vi "Logging Message Loop.vi"(8 "error in (no error)":errorcluster, 9 "Data Notifiers":T1, 10 "Data Queue":refnum<queue>, 11 "Message Queues":T2) -> (0 "error out":errorcluster)   [LabVIEW 2013, in "Logging.lvlib"]
doc: "The message loop subVI to handle messages pertaining to logging data."
uses:
  Logging.lvlib
  support/Message Queue/All Message Queues.ctl
  support/Message Queue/Message Cluster.ctl
  support/Data Notifiers/All Data Notifiers.ctl
  Acquisition/APD Notifier Cluster.ctl
  Piezo/Piezo display.ctl
  XY/XY Display.ctl
  Capacitive/Capacitive Signal Cluster.ctl
  Feedback/Error Signal.ctl
  Logging Configuration.ctl
  Logging State.ctl
  support/Message Queue/Enqueue Message (Single).vi
  <vilib>/Utility/error.llb/Error Cluster From Error Code.vi
  <vilib>/ErrorRing/Error Ring.xnode
  support/Message Queue/Message Queue.lvlib
  Piezo/Piezo.lvlib
  Acquisition/Acquisition.lvlib
  XY/XY.lvlib
  support/Data Notifiers/Data Notifiers.lvlib
  Capacitive/Capacitive.lvlib
  Feedback/Feedback.lvlib
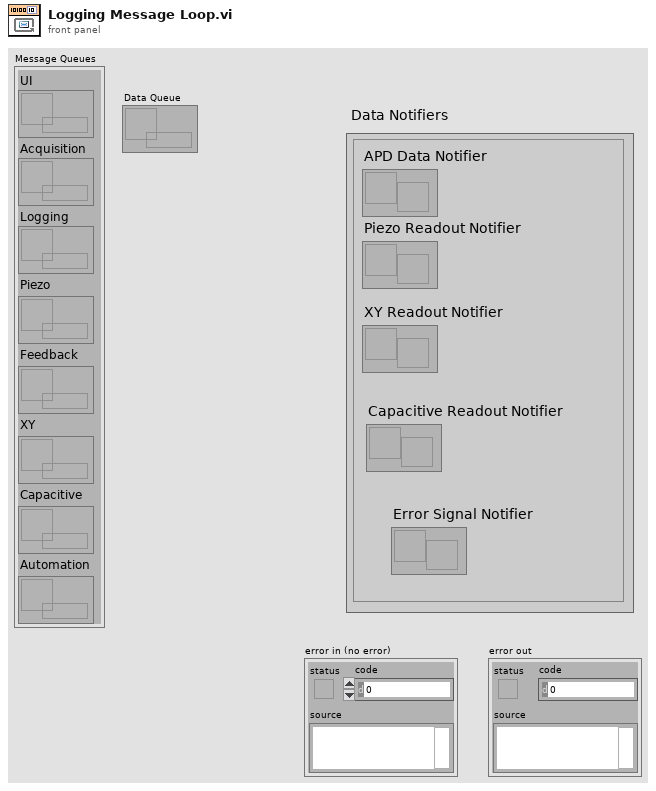
[diagram p1: front panel]
types:
  T1 = typedef "Data Notifiers.lvlib/All Data Notifiers.ctl" = cluster{"APD Data Notifier":refnum<notifier>, "Piezo Readout Notifier":refnum<notifier>, "XY Readout Notifier":refnum<notifier>, "Capacitive Readout Notifier":refnum<notifier>, "Error Signal Notifier":refnum<notifier>}
  T2 = typedef "Message Queue.lvlib/All Message Queues.ctl" = cluster{"UI":refnum<queue>, "Acquisition":refnum<queue>, "Logging":refnum<queue>, "Piezo":refnum<queue>, "Feedback":refnum<queue>, "XY":refnum<queue>, "Capacitive":refnum<queue>, "Automation":refnum<queue>}
  T3 = typedef "Logging.lvlib/Logging State.ctl" = cluster{"State":enum16{"Logging", "Not Logging"}, "Samples to Save":u32, "Start Time":dbl}
  T4 = typedef "Logging.lvlib/Logging Configuration.ctl" = cluster{"Log File Base Path":path, "Max Samples":u32, "File Refnum":refnum<file>, "Log Piezo":bool, "Piezo File Refnum":refnum<file>, "Log Capacitive":bool, "Cap File Refnum":refnum<file>, "Filename":string, "Path where to save":path}
  T5 = cluster{"Value":bool, "Filename":string, "Max. Samp":i32}
  T6 = typedef "Piezo.lvlib/Piezo display.ctl" = cluster{"PiezoPosition":sgl, "Counter Time":i32}
  T7 = typedef "Capacitive.lvlib/Capacitive Signal Cluster.ctl" = cluster{"Readout":sgl, "Time":i32, "Temperature":dbl}
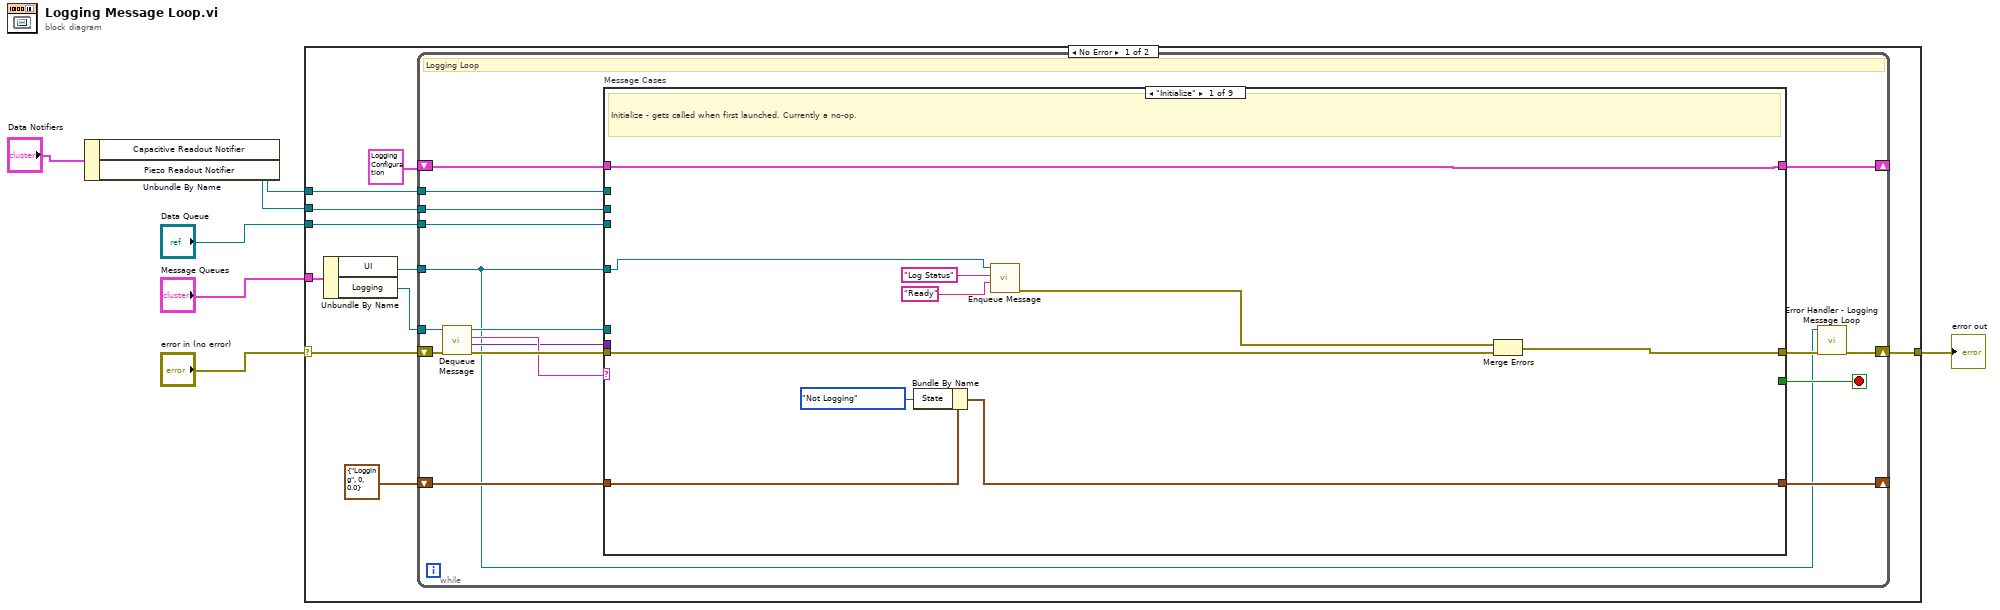
[diagram p0: block diagram]
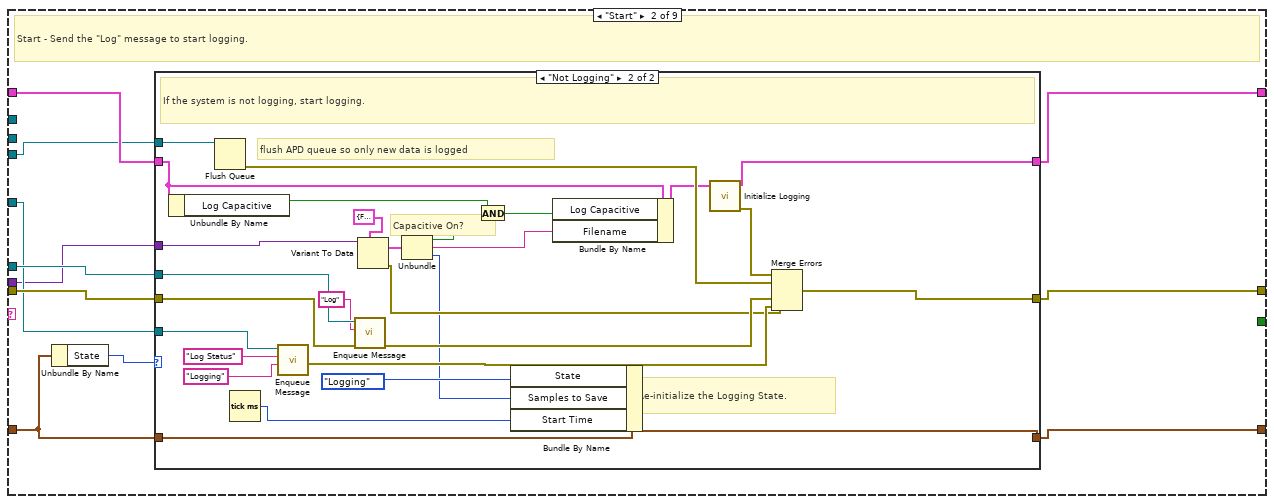
[diagram p2: hidden frame]
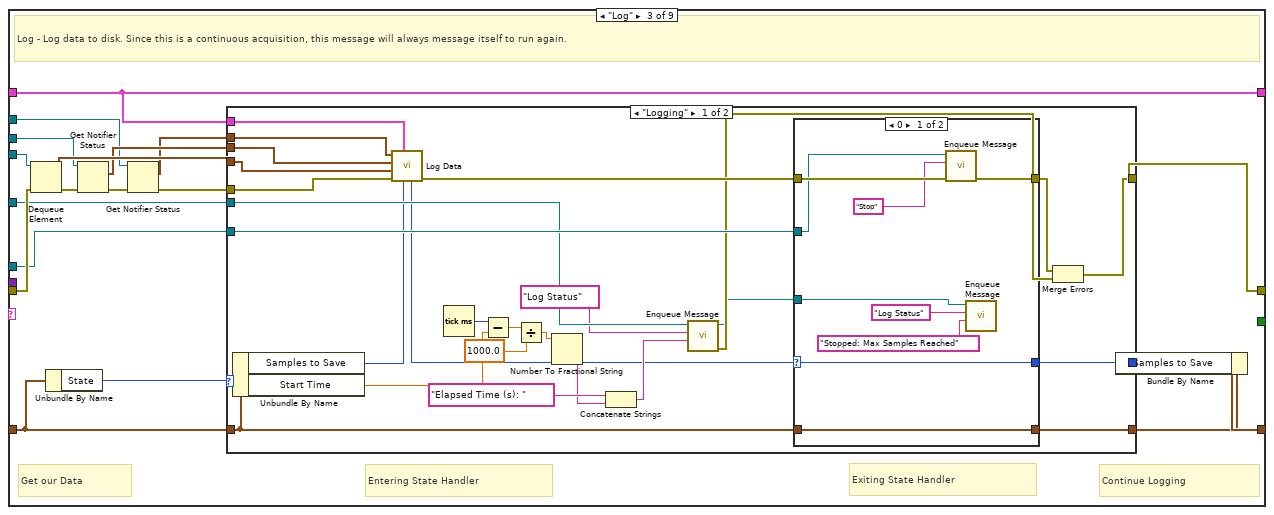
[diagram p4: hidden frame]
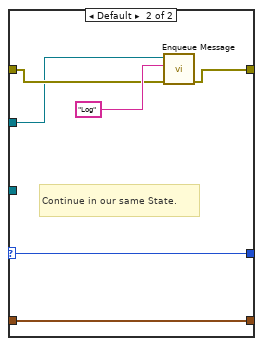
[diagram p5: hidden frame]
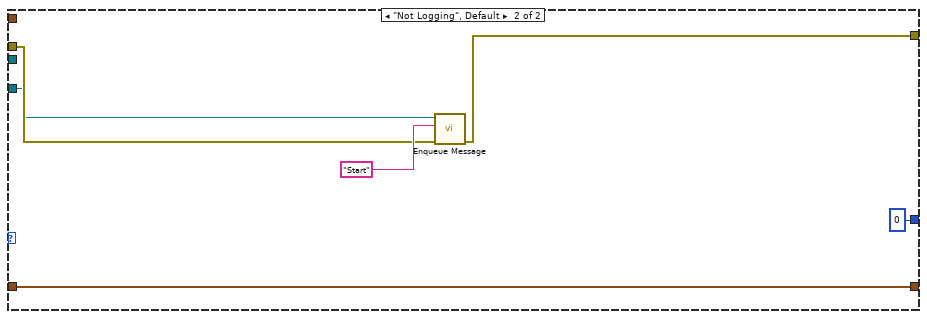
[diagram p6: hidden frame]
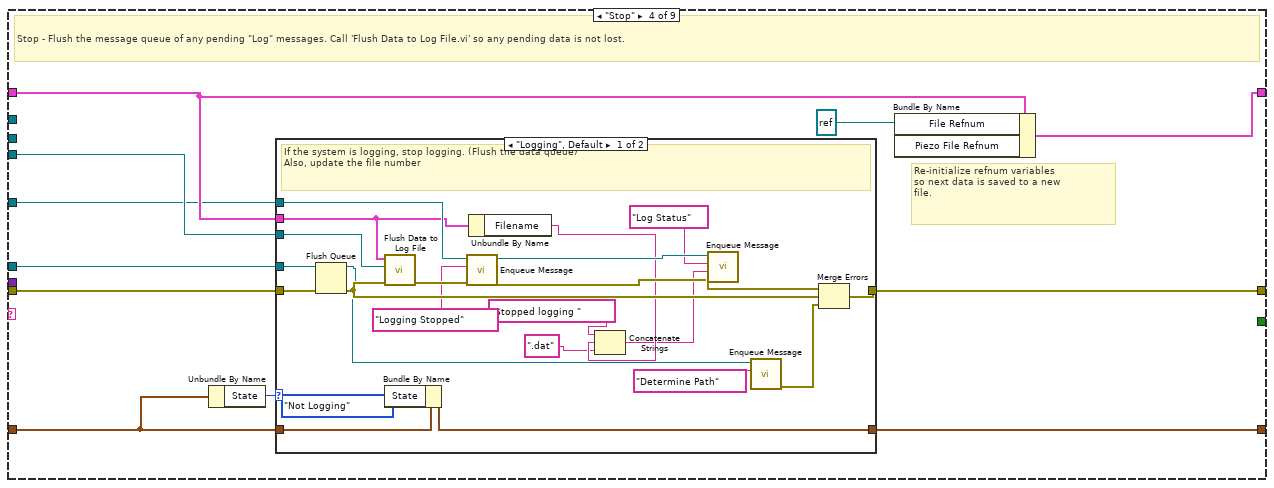
[diagram p7: hidden frame]
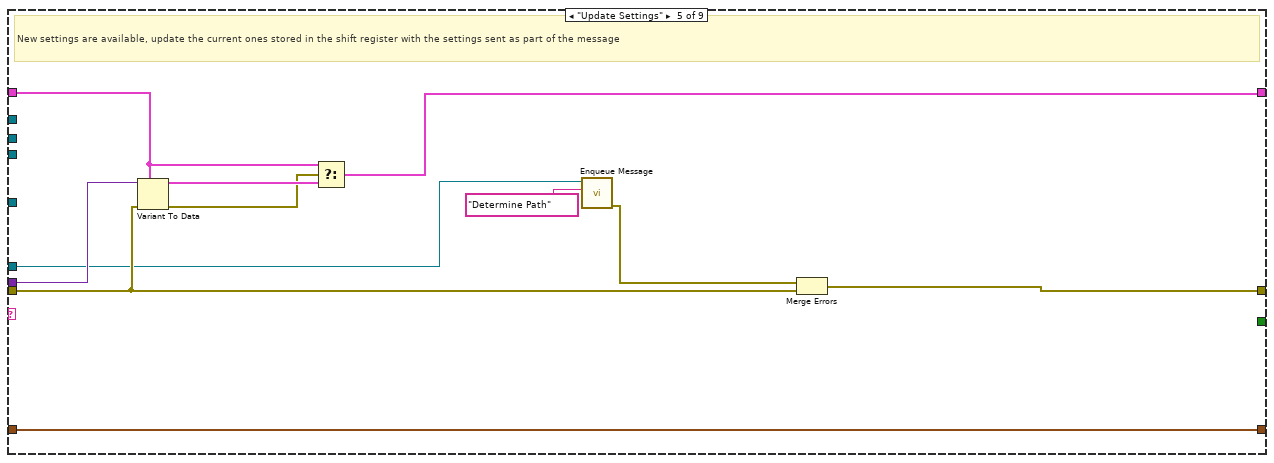
[diagram p9: hidden frame]
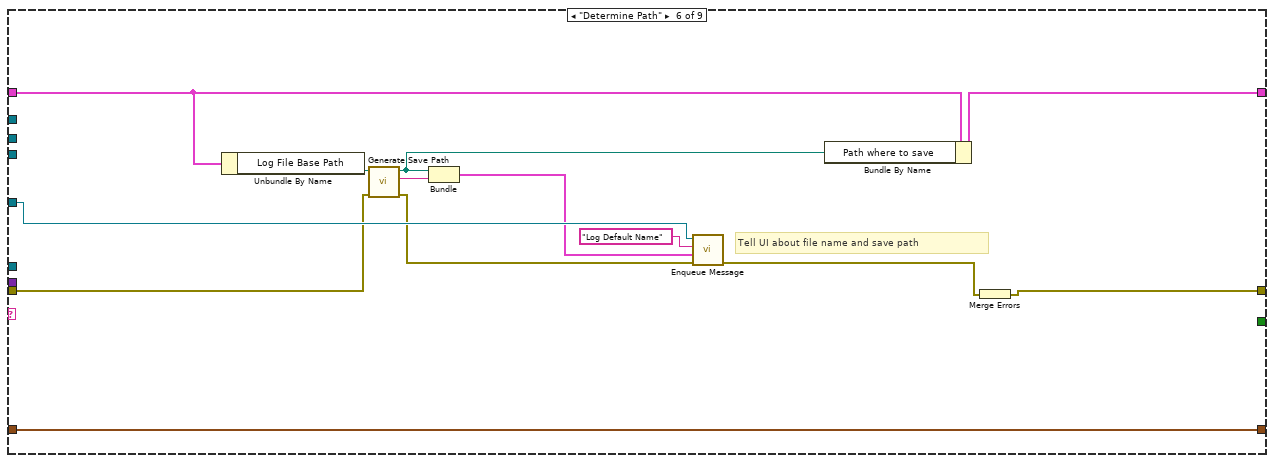
[diagram p10: hidden frame]
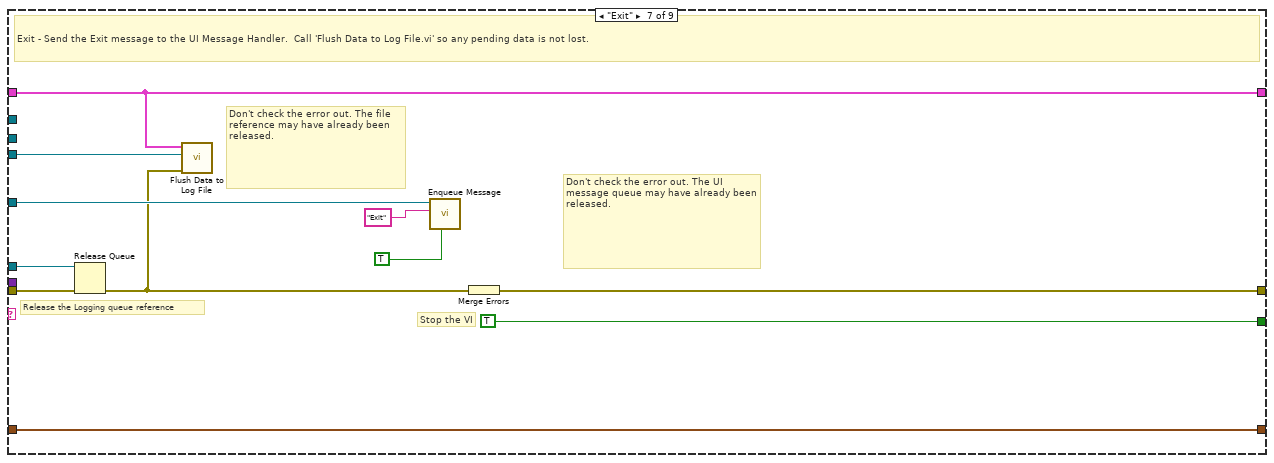
[diagram p11: hidden frame]
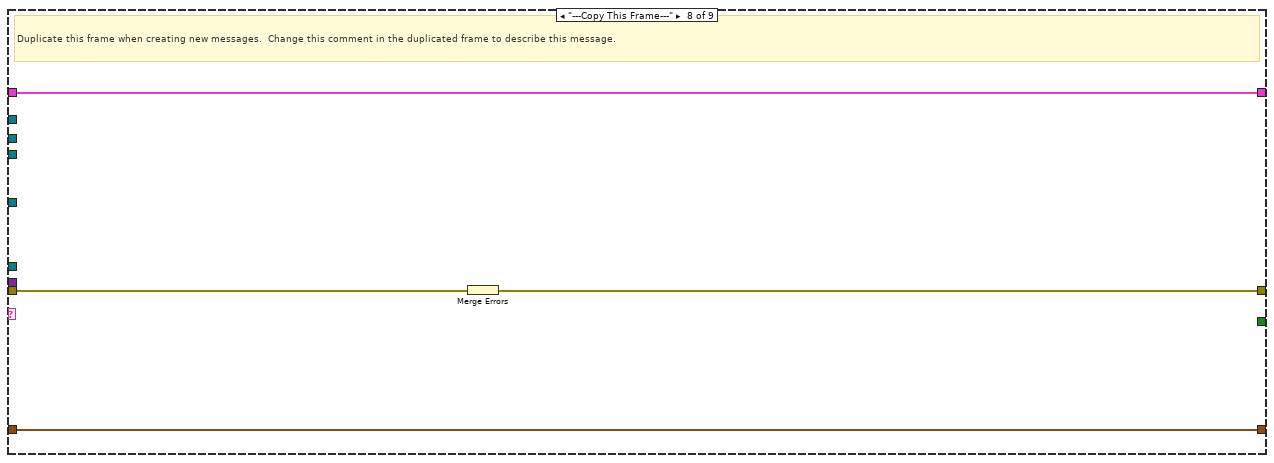
[diagram p12: hidden frame]
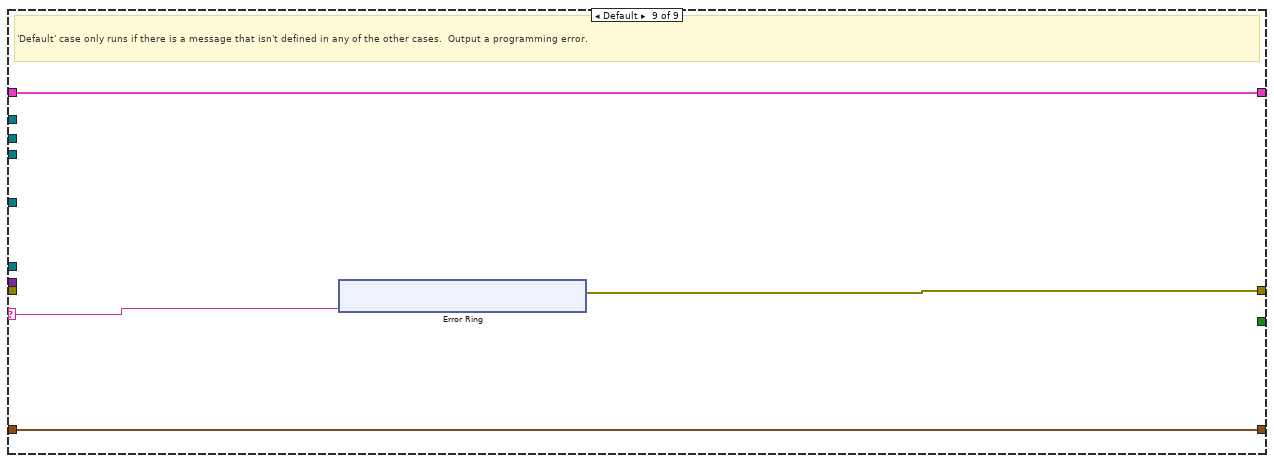
[diagram p13: hidden frame]
diagram:
  n1 = Unbundle By Name("Data Notifiers") -> ("Capacitive Readout Notifier"=w1:refnum<notifier>, "Piezo Readout Notifier"=w2:refnum<notifier>)
  n2 = case shown="No Error" "error in (no error)" {
    selector: "error in (no error)" -> [w13 w239]
    tunnel: "Message Queues" -> [w17 _]
    tunnel: [w15 w239] -> w6
    tunnel: "Data Queue" -> [w12 _]
    tunnel: w2 -> [w9 _]
    tunnel: w1 -> [w8 _]
    frame No Error {
      n3 = Unbundle By Name(w17) -> ("UI"=w11:refnum<queue>, "Logging"=w16:refnum<queue>)
      n4 = while {
        tunnel: w16 -> [w26]
        shift-right: [w33] -> _
        shift-left: T4 {"Log File Base Path"=path "", "Max Samples"=0, "File Refnum"=refnum, "Log Piezo"=FALSE, "Piezo File Refnum"=refnum, "Log Capacitive"=FALSE, "Cap File Refnum"=refnum, "Filename"="", "Path where to save"=path ""} ("Logging Configuration") -> [w34]
        shift-right: [w21] -> w15
        shift-left: w13 -> [w31]
        tunnel: w11 -> [w20]
        tunnel: w12 -> [w25]
        shift-right: [w23] -> _
        shift-left: T3 {"State"=enum."Logging", "Samples to Save"=0, "Start Time"=0.0} -> [w24]
        tunnel: w9 -> [w19]
        tunnel: w8 -> [w18]
        stop <- w32 stop-if-true
        # "Logging Loop"
        n5 = call "Dequeue Message.vi"("error in (no error)"=w31, "Message Queue"=w26) -> ("error out"=w30:errorcluster, "Message Data"=w28:variant, "Message"=w29:string, "dup Message Queue"=w27:refnum<queue>)  [unwired: 6 in]
        n6 = case "Message Cases" shown="\"Initialize\"" w29 {
          selector: w29 -> [_ _ _ _ _ _ _ _ w228]
          tunnel: w27 -> [_ w54 w95 w161 w191 _ w217 _ _]
          tunnel: w30 -> [w43 w53 w105 w162 w193 w202 w220 w227 _]
          tunnel: [w44 w55 w94 w163 w199 w204 w222 w225 w229] -> w22
          tunnel: w34 -> [w36 w52 w101 w159 w197 w207 w216 w226 w231]
          tunnel: [w36 w51 w101 w160 w194 w208 w216 w226 w231] -> w33
          tunnel: [_ _ _ _ _ _ TRUE _ _] -> w32
          tunnel: w28 -> [_ w45 _ _ w198 _ _ _ _]
          tunnel: w20 -> [w37 w47 w100 w157 _ w206 w221 _ _]
          tunnel: w25 -> [_ w46 w98 w158 _ _ w215 _ _]
          tunnel: w24 -> [w42 w49 w103 w155 w192 w200 w213 w224 w230]
          tunnel: [w41 w50 w99 w154 w192 w200 w213 w224 w230] -> w23
          tunnel: w19 -> [_ _ w93 _ _ _ _ _ _]
          tunnel: w18 -> [_ _ w87 _ _ _ _ _ _]
          frame "Initialize" {
            # "Initialize - gets called when first launched. Currently a no-op."
            n7 = Bundle By Name(cluster=w42, "State"=enum16{"Logging", "Not Logging"}."Not Logging") -> (w41:T3)
            n8 = call-poly "Enqueue Message.vi"("Message Data"="Ready" ("Message"), "Message"="Log Status", "Message Queue"=w37) -> ("error out"=w35:errorcluster)  [unwired: 7 in, 1 out]
            n9 = Merge Errors(w35, w43) -> (w44:errorcluster)
          }
          frame "Start" {
            # "Start - Send the \"Log\" message to start logging."
            n10 = Unbundle By Name(w49) -> ("State"=w48:enum16{"Logging", "Not Logging"})
            n11 = case shown="\"Not Logging\"" w48 {
              tunnel: [w57 w80] -> w55
              tunnel: w54 -> [_ w86]
              tunnel: w53 -> [w57 w84]
              tunnel: w52 -> [w58 w70]
              tunnel: [w58 w73] -> w51
              tunnel: w49 -> [w56 w83]
              tunnel: [w56 w82] -> w50
              tunnel: w47 -> [_ w78]
              tunnel: w46 -> [_ w72]
              tunnel: w45 -> [_ w67]
              frame "Logging", Default {
                # "The system is already running. Ignore the \"Start\" message."
              }
              frame "Not Logging" {
                # "Capacitive On?"
                # "flush APD queue so only new data is logged"
                # "Re-initialize the Logging State."
                # "If the system is not logging, start logging."
                n12 = Unbundle By Name(w70) -> ("Log Capacitive"=w68:bool)
                n13 = Flush Queue(queue=w72) -> (error out=w71:errorcluster)  [unwired: 1 in, 2 out]
                n14 = Tick Count (ms)() -> (millisecond timer value=w76:u32)
                n15 = call-poly "Enqueue Message.vi"("Message Data"="Logging" ("Message"), "Message"="Log Status", "Message Queue"=w78) -> ("error out"=w75:errorcluster)  [unwired: 7 in, 1 out]
                n16 = call-poly "Enqueue Message.vi"("error in (no error)"=w84, "Message"="Log", "Message Queue"=w86) -> ("error out"=w74:errorcluster)  [unwired: 7 in, 1 out]
                n17 = Variant To Data(type=T5 {"Value"=FALSE, "Filename"="", "Max. Samp"=0} ("output cluster"), Variant=w67) -> (data=w63:T5, error out=w65:errorcluster)  [unwired: 1 in]
                n18 = Unbundle(w63) -> ("Value"=w62:bool, "Filename"=w61:string, "Max. Samp"=w59:i32)
                n19 = And(x=w68, y=w62) -> (x .and. y?=w64:bool)
                n20 = Bundle By Name(cluster=w83, "State"=enum16{"Logging", "Not Logging"}."Logging", "Samples to Save"=w59, "Start Time"=w76) -> (w82:T3)
                n21 = Bundle By Name(cluster=w70, "Log Capacitive"=w64, "Filename"=w61) -> (w69:T4)
                n22 = call "Initialize Logging.vi"("Logging Configuration"=w69) -> ("error out"=w66:errorcluster, "Logging Configuration Out"=w73:T4)  [unwired: 9 in]
                n23 = Merge Errors(w66, w71, w65, w74, w75) -> (w80:errorcluster)
              }
            }
          }
          frame "Log" {
            # "Exiting State Handler"
            # "Continue Logging"
            # "Entering State Handler"
            # "Get our Data"
            # "Log - Log data to disk. Since this is a continuous acquisition, this message will always message itself to run again."
            n24 = Dequeue Element(queue=w98, error in (no error)=w105) -> (element=w102:waveform(dbl)[], error out=w91:errorcluster)  [unwired: 1 in, 2 out]
            n25 = Unbundle By Name(w103) -> ("State"=w104:enum16{"Logging", "Not Logging"})
            n26 = Get Notifier Status(notifier=w93, error in (no error)=w91) -> (current notification=w92:T6, error out=w90:errorcluster)  [unwired: 3 out]
            n27 = Get Notifier Status(notifier=w87, error in (no error)=w90) -> (current notification=w88:T7, error out=w89:errorcluster)  [unwired: 3 out]
            n28 = case shown="\"Logging\"" w104 {
              tunnel: [w129 w149] -> w97
              tunnel: w103 -> [w130 w149]
              tunnel: w102 -> [w109 _]
              tunnel: w89 -> [w131 w151]
              tunnel: w101 -> [w107 _]
              tunnel: w100 -> [w121 _]
              tunnel: [w113 w147] -> w94
              tunnel: [w128 0] -> w96
              tunnel: w95 -> [w126 w150]
              tunnel: w92 -> [w108 _]
              tunnel: w88 -> [w106 _]
              frame "Logging" {
                n29 = Unbundle By Name(w130) -> ("Samples to Save"=w111:u32, "Start Time"=w124:dbl)
                n30 = call "Log Data.vi"("Samples to Save In"=w111, "Logging Configuration"=w107, "error in (no error)"=w131, "Data"=w109, "Piezo Data"=w108, "Cap Data"=w106) -> ("error out"=w127:errorcluster, "Samples to Save Out"=w110:u32)  [unwired: 4 in]
                n31 = Tick Count (ms)() -> (millisecond timer value=w125:u32)
                n32 = Subtract(x=w125, y=w124) -> (x-y=w123:dbl)
                n33 = Divide(x=w123, y=1000.0) -> (x/y=w119:dbl)
                n34 = Number To Fractional String(number=w119) -> (F-format string=w117:string)  [unwired: 3 in]
                n35 = Concatenate Strings("Elapsed Time (s): " ("Message"), w117) -> (w116:string)
                n36 = call-poly "Enqueue Message.vi"("Message Data"=w116, "Message"="Log Status", "Message Queue"=w121) -> ("error out"=w114:errorcluster, "dup Message Queue"=w112:refnum<queue>)  [unwired: 7 in]
                n37 = case shown="0" w110 {
                  selector: w110 -> [w140 w146]
                  tunnel: w127 -> [w138 w143]
                  tunnel: [w139 w142] -> w115
                  tunnel: w130 -> [w132 w145]
                  tunnel: [w132 w145] -> w129
                  tunnel: [w140 w146] -> w128
                  tunnel: w126 -> [w136 w141]
                  tunnel: w112 -> [w133 _]
                  frame 0 {
                    n38 = call-poly "Enqueue Message.vi"("error in (no error)"=w138, "Message"="Stop", "Message Queue"=w136) -> ("error out"=w139:errorcluster)  [unwired: 7 in, 1 out]
                    n39 = call-poly "Enqueue Message.vi"("Message Data"="Stopped: Max Samples Reached" ("Message"), "Message"="Log Status", "Message Queue"=w133) -> ()  [unwired: 7 in, 2 out]
                  }
                  frame Default {
                    # "Continue in our same State."
                    n40 = call-poly "Enqueue Message.vi"("error in (no error)"=w143, "Message"="Log", "Message Queue"=w141) -> ("error out"=w142:errorcluster)  [unwired: 7 in, 1 out]
                  }
                }
                n41 = Merge Errors(w115, w114) -> (w113:errorcluster)
              }
              frame "Not Logging", Default {
                n42 = call-poly "Enqueue Message.vi"("error in (no error)"=w151, "Message"="Start", "Message Queue"=w150) -> ("error out"=w147:errorcluster)  [unwired: 7 in, 1 out]
              }
            }
            n43 = Bundle By Name(cluster=w97, "Samples to Save"=w96) -> (w99:T3)
          }
          frame "Stop" {
            w153 = refnum<file> refnum ("File Refnum")
            # "Re-initialize refnum variables\nso next data is saved to a new\nfile."
            # "Stop - Flush the message queue of any pending \"Log\" messages. Call 'Flush Data to Log File.vi' so any pending data is not lost."
            n44 = Unbundle By Name(w155) -> ("State"=w156:enum16{"Logging", "Not Logging"})
            n45 = case shown="\"Logging\", Default" w156 {
              tunnel: [w186 w188] -> w163
              tunnel: w162 -> [w185 w188]
              tunnel: w161 -> [w184 _]
              tunnel: w159 -> [w168 _]
              tunnel: w158 -> [w183 _]
              tunnel: w157 -> [w180 _]
              tunnel: w155 -> [w178 w187]
              tunnel: [w177 w187] -> w154
              frame "Logging", Default {
                # "If the system is logging, stop logging. (Flush the data queue)\nAlso, update the file number"
                n46 = Flush Queue(queue=w184, error in (no error)=w185) -> (queue out=w171:refnum<queue>, error out=w182:errorcluster)  [unwired: 1 out]
                n47 = call "Flush Data to Log File.vi"("error in (no error)"=w182, "Data Queue"=w183, "Logging Configuration"=w168) -> ("error out"=w181:errorcluster)  [unwired: 8 in]
                n48 = Bundle By Name(cluster=w178, "State"=enum16{"Logging", "Not Logging", "Idle"}."Not Logging") -> (w177:T3)
                n49 = call-poly "Enqueue Message.vi"("error in (no error)"=w181, "Message"="Logging Stopped", "Message Queue"=w180) -> ("error out"=w174:errorcluster, "dup Message Queue"=w173:refnum<queue>)  [unwired: 7 in]
                n50 = Unbundle By Name(w168) -> ("Filename"=w166:string)
                n51 = Concatenate Strings("Stopped logging " ("Message"), w166, ".dat" ("Message")) -> (w164:string)
                n52 = call-poly "Enqueue Message.vi"("error in (no error)"=w174, "Message Data"=w164, "Message"="Log Status", "Message Queue"=w173) -> ("error out"=w175:errorcluster)  [unwired: 6 in, 1 out]
                n53 = call-poly "Enqueue Message.vi"("Message"="Determine Path", "Message Queue"=w171) -> ("error out"=w169:errorcluster)  [unwired: 8 in, 1 out]
                n54 = Merge Errors(w175, w182, w169) -> (w186:errorcluster)
              }
              frame "Not Logging" {
                # "The system is already idle. Ignore the \"Stop\" message."
              }
            }
            n55 = Bundle By Name(cluster=w159, "File Refnum"=w153, "Piezo File Refnum"=w153) -> (w160:T4)
          }
          frame "Update Settings" {
            # "New settings are available, update the current ones stored in the shift register with the settings sent as part of the message"
            n56 = Variant To Data(error in=w193, type=w197, Variant=w198) -> (data=w196:T4, error out=w195:errorcluster)
            n57 = Select(t=w197, s=w195, f=w196) -> (s? t:f=w194:T4)
            n58 = call-poly "Enqueue Message.vi"("Message"="Determine Path", "Message Queue"=w191) -> ("error out"=w190:errorcluster)  [unwired: 8 in, 1 out]
            n59 = Merge Errors(w190, w193) -> (w199:errorcluster)
          }
          frame "Determine Path" {
            # "Tell UI about file name and save path"
            n60 = Unbundle By Name(w207) -> ("Log File Base Path"=w211:path)
            n61 = call "Generate Save Path.vi"("error in (no error)"=w202, "Log File Base Path"=w211) -> ("error out"=w201:errorcluster, "Save String"=w210:string, "Save Path"=w209:path)  [unwired: 7 in]
            n62 = Bundle("Save Path"=w209, "Save String"=w210) -> (w205:cluster{"Save Path":path, "Save String":string})  [unwired: 1 in]
            n63 = call-poly "Enqueue Message.vi"("error in (no error)"=w201, "Message Data"=w205, "Message"="Log Default Name", "Message Queue"=w206) -> ("error out"=w203:errorcluster)  [unwired: 6 in, 1 out]
            n64 = Bundle By Name(cluster=w207, "Path where to save"=w209) -> (w208:T4)
            n65 = Merge Errors(w203) -> (w204:errorcluster)
          }
          frame "Exit" {
            # "Don't check the error out. The file reference may have already been released."
            # "Release the Logging queue reference"
            # "Don't check the error out. The UI message queue may have already been released."
            # "Stop the VI"
            # "Exit - Send the Exit message to the UI Message Handler.  Call 'Flush Data to Log File.vi' so any pending data is not lost."
            n66 = Release Queue(queue=w217, error in (no error)=w220) -> (error out=w214:errorcluster)  [unwired: 1 in, 2 out]
            n67 = call "Flush Data to Log File.vi"("error in (no error)"=w214, "Data Queue"=w215, "Logging Configuration"=w216) -> ()  [unwired: 8 in, 1 out]
            n68 = call-poly "Enqueue Message.vi"("Priority Message? (F)"=TRUE, "Message"="Exit", "Message Queue"=w221) -> ()  [unwired: 7 in, 2 out]
            n69 = Merge Errors(w214) -> (w222:errorcluster)
          }
          frame "---Copy This Frame---" {
            # "Duplicate this frame when creating new messages.  Change this comment in the duplicated frame to describe this message."
            n70 = Merge Errors(w227) -> (w225:errorcluster)
          }
          frame Default {
            # "'Default' case only runs if there is a message that isn't defined in any of the other cases.  Output a programming error."
            n71 = xnode "Error Ring"("parameter 0"=w228) -> ("error out"=w229:errorcluster)
          }
        }
        n72 = call "Error Handler - Logging Message Loop.vi"("error in (no error)"=w22, "Message Queue"=w20) -> ("dup error in"=w21:errorcluster)  [unwired: 8 in, 1 out]
      }
    }
    frame Error {
    }
  }
  "error out" <- w6
